vi "Reserve Memory and Read CalibrConst from CnfgFile.vi"(3 "error out 2":errorcluster, 4 "pathCalibrConsts":path, 5 "pathConfigFile":path) -> (0 "error out":errorcluster, 1 "Master or Slave?":T1[](array[typedef]))   [LabVIEW 2009, in "POLARIS BME DG.lvlib" / "BME_DG_System.lvclass"]
uses:
  BME_DG_System.lvclass
  LV-BME Interface/BME_DG_MasterOrSlave.ctl
  POLARIS BME DG.lvlib
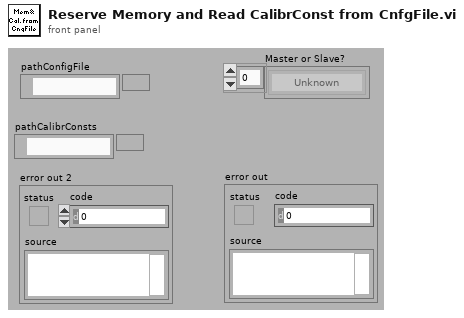
[diagram p1: front panel]
types:
  T1 = typedef "POLARIS BME DG.lvlib/BME_DG_MasterOrSlave.ctl" = enum16{"Unknown", "Master", "Slave"}
  T2 = typedef "POLARIS BME DG.lvlib/DetectDG.ctl" = cluster{"DG_Number":i32, "DG_Product":i32, "Product Name":string, "Bus_Number":i32, "Slot_Number":i32, "Master":bool}
  T3 = typedef "POLARIS BME DG.lvlib/System DG Selection.ctl" = cluster{"Selected System DGs":T2[], "Name":string}
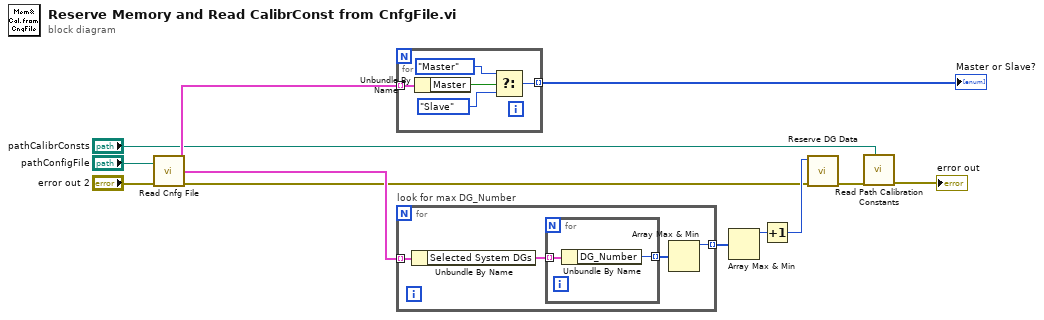
[diagram p0: block diagram]
diagram:
  n1 = call "Read Cnfg File.vi"("Config File"="pathConfigFile", "error in (no error)"="error out 2") -> ("InstalledDGs"=w11:T2[], "DGSystems"=w4:T3[], "error out"=w3:errorcluster)  [unwired: 8 in, 3 out]
  n2 = for {
    tunnel: w11 -> [w17] mode=indexing
    tunnel: [w13] -> w12 mode=indexing
    n3 = Unbundle By Name(w17) -> ("Master"=w16:bool)
    n4 = Select(t=BME_DG_MasterOrSlave."Master", s=w16, f=BME_DG_MasterOrSlave."Slave") -> (s? t:f=w13:T1)
  }
  "Master or Slave?" <- w12
  n5 = for "look for max DG_Number" {
    tunnel: w4 -> [w21] mode=indexing
    tunnel: [w18] -> w10 mode=indexing
    n6 = Unbundle By Name(w21) -> ("Selected System DGs"=w20:T2[])
    n7 = for {
      tunnel: w20 -> [w22] mode=indexing
      tunnel: [w23] -> w19 mode=indexing
      n8 = Unbundle By Name(w22) -> ("DG_Number"=w23:i32)
    }
    n9 = Array Max & Min(array=w19) -> (max value=w18:i32)  [unwired: 3 out]
  }
  n10 = Array Max & Min(array=w10) -> (max value=w5:i32)  [unwired: 3 out]
  n11 = Increment(x=w5) -> (x+1=w6:i32)
  n12 = call "Reserve DG Data.vi"("error in (no error)"=w3, "Number Of Delay Generators"=w6) -> ("error out"=w7:errorcluster)  [unwired: 9 in]
  n13 = call "Read Path Calibration Constants.vi"("Path"="pathCalibrConsts", "error in (no error)"=w7) -> ("error out"=→"error out":errorcluster)  [unwired: 9 in]
